vi "example_GInterrupt.vi"() -> ()   [LabVIEW 2020]
uses:
  <vilib>/Galil/resources/gclib32/gclib32.lvlib
  <vilib>/Galil/resources/gclibo32/gclibo32.lvlib
panel:
  out "Interrupt Code":u8
  out "Error Out":errorcluster
  in  "IP Address":string="192.168.1.77 -s EI"
  in  "Command":string="EI 1; SHA; PA 5000; BGA"
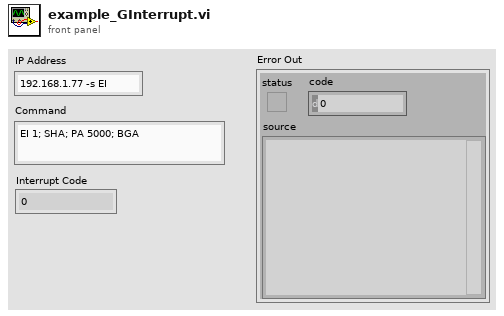
[diagram p1: front panel]
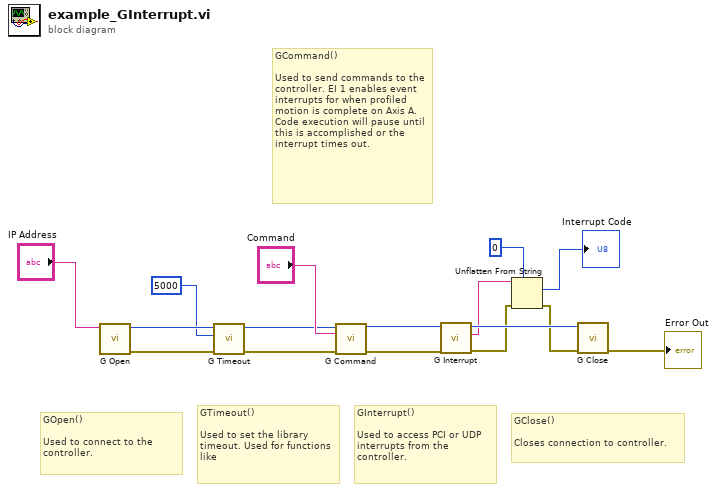
[diagram p0: block diagram]
diagram:
  # "GTimeout()\n\nUsed to set the library timeout. Used for functions like"
  # "GInterrupt()\n\nUsed to access PCI or UDP interrupts from the controller."
  # "GClose()\n\nCloses connection to controller."
  # "GCommand()\n\nUsed to send commands to the controller. EI 1 enables event interrupts for when profiled motion is complete on Axis A. Code execution will pause until this is accomplished or the interrupt times out."
  # "GOpen()\n\nUsed to connect to the controller."
  n1 = call <vilib>:"G Open.vi"("address"="IP Address") -> ("error out"=w1:errorcluster, "g out"=w3:u32)  [unwired: 8 in]
  n2 = call <vilib>:"G Timeout.vi"("error in (no error)"=w1, "timeout_ms"=i16 5000, "g"=w3) -> ("error out"=w5:errorcluster, "g out"=w4:u32)  [unwired: 7 in]
  n3 = call <vilib>:"G Command.vi"("g"=w4, "command"="Command", "error in (no error)"=w5) -> ("g out"=w13:u32, "error out"=w12:errorcluster)  [unwired: 10 in, 1 out]
  n4 = call <vilib>:"G Interrupt.vi"("error in (no error)"=w12, "g"=w13) -> ("error out"=w7:errorcluster, "status_byte out"=w10:string, "g out"=w11:u32)  [unwired: 7 in]
  n5 = Unflatten From String(type=u8 0, binary string=w10, error in (no error)=w7) -> (value=→"Interrupt Code":u8, error out=w6:errorcluster)  [unwired: 2 in, 1 out]
  n6 = call <vilib>:"G Close.vi"("error in (no error)"=w6, "g"=w11) -> ("error out"=→"Error Out":errorcluster)  [unwired: 9 in]
